vi "Turn to Angle.vi"(10 "Target Angle":dbl) -> (2 "Output Rotation":dbl)   [LabVIEW 2016]
uses:
  Drive Globals.vi
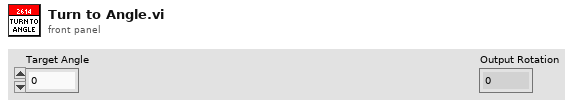
[diagram p1: front panel]
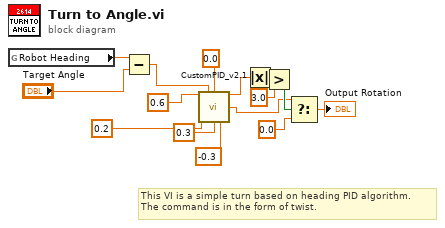
[diagram p0: block diagram]
diagram:
  # "This VI is a simple turn based on heading PID algorithm.\nThe command is in the form of twist."
  n1 = global read "Drive Globals.vi" "Robot Heading"() -> (w5:dbl)
  n2 = Subtract(x=w5, y="Target Angle") -> (x-y=w4:dbl)
  n3 = call "CustomPID_v2.1.vi"("Kp"=0.6, "Process Variable"=w4, "Goal"=0.0, "Kd"=0.2, "Max Ouput"=0.3, "Min Output"=-0.3) -> ("Current Error"=w13:dbl, "Command"=w7:dbl)  [unwired: 7 in, 1 out]
  n4 = Absolute Value(x=w13) -> (abs(x)=w12:dbl)
  n5 = Greater?(x=w12, y=3.0) -> (0:w9:bool)
  n6 = Select(t=w7, s=w9, f=0.0 ("t")) -> (s? t:f=→"Output Rotation":dbl)
